vi "python-similarity.vi"() -> ()   [LabVIEW 2020]
panel:
  out "res out":dbl[](array[numeric])
  in  "diff":dbl=1.2 format="%#_13g"
  in  "data":dbl[][](array[numeric])=[[0.0, 1.0, 0.4, 2.0, 5.0, 1.0, 0.0, 0.0], [5.0, 2.0, 0.45, 2.1, 5.5, 1.0, 0.0, 0.0], [6.0, 0.8, 0.35, 2.0, 1.0, 5.0, 0.0, -1.0]]
  in  "module path":path=path "C:/dev/pyconlyse/utilities/mytests/test1.py"
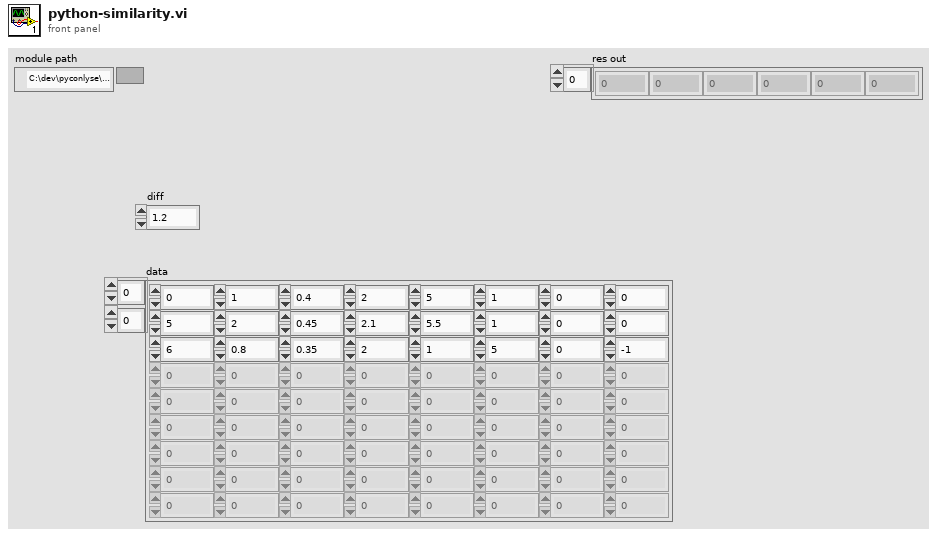
[diagram p1: front panel]
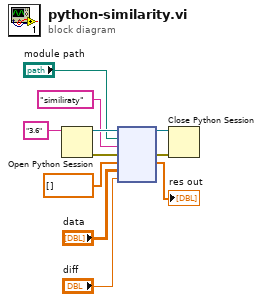
[diagram p0: block diagram]
diagram:
  n1 = Open Python Session(python version="3.6" ("Python version")) -> (session out=w10:refnum<k35>, error out=w7:errorcluster)  [unwired: 2 in]
  n2 = node(w10, "module path", "similiraty" ("function name"), w7, dbl[] [], "data", "diff") -> (w9:refnum<k35>, w6:errorcluster, →"res out":dbl[])  [unwired: 2 in, 2 out]
  n3 = Close Python Session(session in=w9, error in=w6) -> ()  [unwired: 1 out]
